vi "Intialize Shared Variable.vi"(8 "error in (no error)":errorcluster, 11 "Master Configuration":T1) -> (0 "error out":errorcluster)   [LabVIEW 2014]
uses:
  controls/Master Configuration.ctl
  controls/EPICS Configuration.ctl
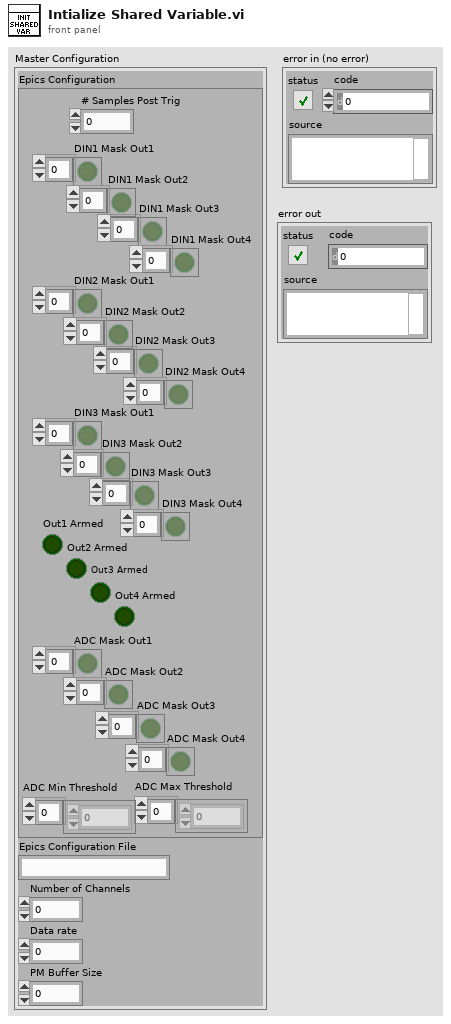
[diagram p1: front panel]
types:
  T1 = typedef "Master Configuration.ctl" = cluster{"Epics Configuration":T2, "Epics Configuration File":string, "Number of Channels":u8, "Data rate":u32, "PM Buffer Size":u32}
  T2 = typedef "EPICS Configuration.ctl" = cluster{"DIN1 Mask Out1":bool[], "# Samples Post Trig":u32, "ADC Mask Out1":bool[], "ADC Max Threshold":dbl[], "ADC Min Threshold":dbl[], "DIN1 Mask Out2":bool[], "DIN1 Mask Out3":bool[], "DIN1 Mask Out4":bool[], "Out3 Armed":bool, "Out1 Armed":bool, "Out4 Armed":bool, "Out2 Armed":bool, "DIN2 Mask Out1":bool[], "DIN2 Mask Out2":bool[], "DIN2 Mask Out3":bool[], "DIN2 Mask Out4":bool[], "DIN3 Mask Out1":bool[], "DIN3 Mask Out2":bool[], "DIN3 Mask Out3":bool[], "DIN3 Mask Out4":bool[], "ADC Mask Out2":bool[], "ADC Mask Out3":bool[], "ADC Mask Out4":bool[]}
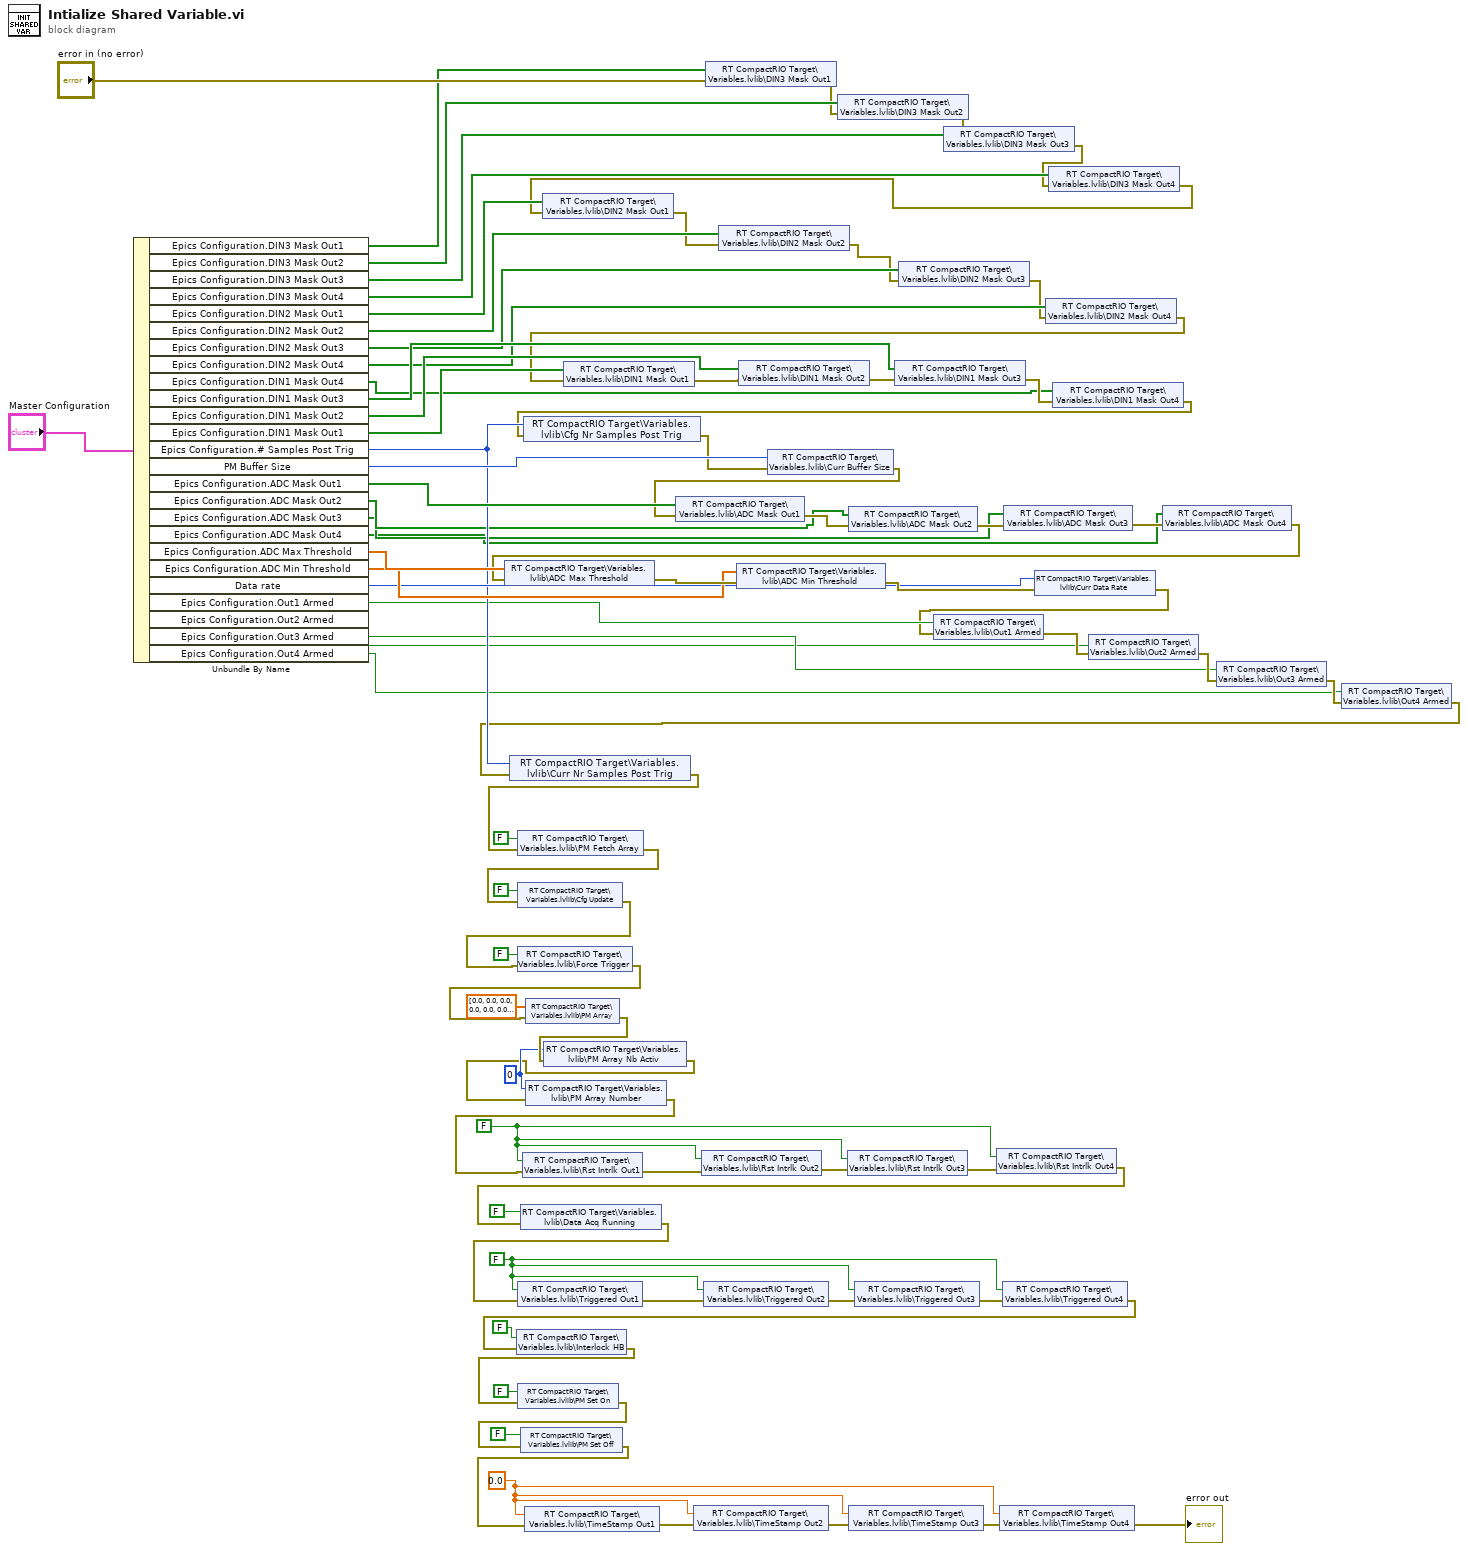
[diagram p0: block diagram]
diagram:
  w39 = 0.0 ("TimeStamp")
  w43 = FALSE ("Triggered")
  w48 = FALSE ("Reset Interlock")
  w2 = u8 0 ("PM Array Number")
  n1 = Unbundle By Name("Master Configuration") -> ("Epics Configuration.DIN3 Mask Out1"=w22:bool[], "Epics Configuration.DIN3 Mask Out2"=w23:bool[], "Epics Configuration.DIN3 Mask Out3"=w24:bool[], "Epics Configuration.DIN3 Mask Out4"=w25:bool[], "Epics Configuration.DIN2 Mask Out1"=w26:bool[], "Epics Configuration.DIN2 Mask Out2"=w27:bool[], "Epics Configuration.DIN2 Mask Out3"=w28:bool[], "Epics Configuration.DIN2 Mask Out4"=w29:bool[], "Epics Configuration.DIN1 Mask Out4"=w53:bool[], "Epics Configuration.DIN1 Mask Out3"=w54:bool[], "Epics Configuration.DIN1 Mask Out2"=w55:bool[], "Epics Configuration.DIN1 Mask Out1"=w79:bool[], "Epics Configuration.# Samples Post Trig"=w62:u32, "PM Buffer Size"=w64:u32, "Epics Configuration.ADC Mask Out1"=w75:bool[], "Epics Configuration.ADC Mask Out2"=w9:bool[], "Epics Configuration.ADC Mask Out3"=w8:bool[], "Epics Configuration.ADC Mask Out4"=w7:bool[], "Epics Configuration.ADC Max Threshold"=w73:dbl[], "Epics Configuration.ADC Min Threshold"=w72:dbl[], "Data rate"=w65:u32, "Epics Configuration.Out1 Armed"=w31:bool, "Epics Configuration.Out2 Armed"=w32:bool, "Epics Configuration.Out3 Armed"=w33:bool, "Epics Configuration.Out4 Armed"=w34:bool)
  n2 = shared-variable "RT CompactRIO Target\\Variables.lvlib\\DIN3 Mask Out1"(w22, error in="error in (no error)") -> (error out=w21:errorcluster)
  n3 = shared-variable "RT CompactRIO Target\\Variables.lvlib\\DIN3 Mask Out2"(w23, error in=w21) -> (error out=w20:errorcluster)
  n4 = shared-variable "RT CompactRIO Target\\Variables.lvlib\\DIN3 Mask Out3"(w24, error in=w20) -> (error out=w19:errorcluster)
  n5 = shared-variable "RT CompactRIO Target\\Variables.lvlib\\DIN3 Mask Out4"(w25, error in=w19) -> (error out=w18:errorcluster)
  n6 = shared-variable "RT CompactRIO Target\\Variables.lvlib\\DIN2 Mask Out1"(w26, error in=w18) -> (error out=w17:errorcluster)
  n7 = shared-variable "RT CompactRIO Target\\Variables.lvlib\\DIN2 Mask Out2"(w27, error in=w17) -> (error out=w16:errorcluster)
  n8 = shared-variable "RT CompactRIO Target\\Variables.lvlib\\DIN2 Mask Out3"(w28, error in=w16) -> (error out=w15:errorcluster)
  n9 = shared-variable "RT CompactRIO Target\\Variables.lvlib\\DIN2 Mask Out4"(w29, error in=w15) -> (error out=w14:errorcluster)
  n10 = shared-variable "RT CompactRIO Target\\Variables.lvlib\\DIN1 Mask Out1"(w79, error in=w14) -> (error out=w57:errorcluster)
  n11 = shared-variable "RT CompactRIO Target\\Variables.lvlib\\DIN1 Mask Out2"(w55, error in=w57) -> (error out=w59:errorcluster)
  n12 = shared-variable "RT CompactRIO Target\\Variables.lvlib\\DIN1 Mask Out3"(w54, error in=w59) -> (error out=w58:errorcluster)
  n13 = shared-variable "RT CompactRIO Target\\Variables.lvlib\\DIN1 Mask Out4"(w53, error in=w58) -> (error out=w56:errorcluster)
  n14 = shared-variable "RT CompactRIO Target\\Variables.lvlib\\Cfg Nr Samples Post Trig"(w62, error in=w56) -> (error out=w63:errorcluster)
  n15 = shared-variable "RT CompactRIO Target\\Variables.lvlib\\Curr Buffer Size"(w64, error in=w63) -> (error out=w4:errorcluster)
  n16 = shared-variable "RT CompactRIO Target\\Variables.lvlib\\ADC Mask Out1"(w75, error in=w4) -> (error out=w10:errorcluster)
  n17 = shared-variable "RT CompactRIO Target\\Variables.lvlib\\ADC Mask Out2"(w9, error in=w10) -> (error out=w13:errorcluster)
  n18 = shared-variable "RT CompactRIO Target\\Variables.lvlib\\ADC Mask Out3"(w8, error in=w13) -> (error out=w12:errorcluster)
  n19 = shared-variable "RT CompactRIO Target\\Variables.lvlib\\ADC Mask Out4"(w7, error in=w12) -> (error out=w11:errorcluster)
  n20 = shared-variable "RT CompactRIO Target\\Variables.lvlib\\ADC Max Threshold"(w73, error in=w11) -> (error out=w74:errorcluster)
  n21 = shared-variable "RT CompactRIO Target\\Variables.lvlib\\ADC Min Threshold"(w72, error in=w74) -> (error out=w71:errorcluster)
  n22 = shared-variable "RT CompactRIO Target\\Variables.lvlib\\Curr Data Rate"(w65, error in=w71) -> (error out=w5:errorcluster)
  n23 = shared-variable "RT CompactRIO Target\\Variables.lvlib\\Out1 Armed"(w31, error in=w5) -> (error out=w37:errorcluster)
  n24 = shared-variable "RT CompactRIO Target\\Variables.lvlib\\Out2 Armed"(w32, error in=w37) -> (error out=w36:errorcluster)
  n25 = shared-variable "RT CompactRIO Target\\Variables.lvlib\\Out3 Armed"(w33, error in=w36) -> (error out=w35:errorcluster)
  n26 = shared-variable "RT CompactRIO Target\\Variables.lvlib\\Out4 Armed"(w34, error in=w35) -> (error out=w6:errorcluster)
  n27 = shared-variable "RT CompactRIO Target\\Variables.lvlib\\Curr Nr Samples Post Trig"(w62, error in=w6) -> (error out=w61:errorcluster)
  n28 = shared-variable "RT CompactRIO Target\\Variables.lvlib\\PM Fetch Array"(FALSE ("PM Fetch Array"), error in=w61) -> (error out=w86:errorcluster)
  n29 = shared-variable "RT CompactRIO Target\\Variables.lvlib\\Cfg Update"(FALSE ("Cfg Update"), error in=w86) -> (error out=w83:errorcluster)
  n30 = shared-variable "RT CompactRIO Target\\Variables.lvlib\\Force Trigger"(FALSE ("Force Trigger"), error in=w83) -> (error out=w82:errorcluster)
  n31 = shared-variable "RT CompactRIO Target\\Variables.lvlib\\PM Array"(sgl[] [0.0, 0.0, 0.0, 0.0, 0.0, 0.0, 0.0, 0.0, 0.0, 0.0, 0.0, 0.0, 0.0, 0.0, 0.0, 0.0] ("PM Array"), error in=w82) -> (error out=w3:errorcluster)
  n32 = shared-variable "RT CompactRIO Target\\Variables.lvlib\\PM Array Nb Activ"(w2, error in=w3) -> (error out=w1:errorcluster)
  n33 = shared-variable "RT CompactRIO Target\\Variables.lvlib\\PM Array Number"(w2, error in=w1) -> (error out=w60:errorcluster)
  n34 = shared-variable "RT CompactRIO Target\\Variables.lvlib\\Rst Intrlk Out1"(w48, error in=w60) -> (error out=w50:errorcluster)
  n35 = shared-variable "RT CompactRIO Target\\Variables.lvlib\\Rst Intrlk Out2"(w48, error in=w50) -> (error out=w52:errorcluster)
  n36 = shared-variable "RT CompactRIO Target\\Variables.lvlib\\Rst Intrlk Out3"(w48, error in=w52) -> (error out=w51:errorcluster)
  n37 = shared-variable "RT CompactRIO Target\\Variables.lvlib\\Rst Intrlk Out4"(w48, error in=w51) -> (error out=w49:errorcluster)
  n38 = shared-variable "RT CompactRIO Target\\Variables.lvlib\\Data Acq Running"(FALSE ("Reset Interlock"), error in=w49) -> (error out=w77:errorcluster)
  n39 = shared-variable "RT CompactRIO Target\\Variables.lvlib\\Triggered Out1"(w43, error in=w77) -> (error out=w45:errorcluster)
  n40 = shared-variable "RT CompactRIO Target\\Variables.lvlib\\Triggered Out2"(w43, error in=w45) -> (error out=w47:errorcluster)
  n41 = shared-variable "RT CompactRIO Target\\Variables.lvlib\\Triggered Out3"(w43, error in=w47) -> (error out=w46:errorcluster)
  n42 = shared-variable "RT CompactRIO Target\\Variables.lvlib\\Triggered Out4"(w43, error in=w46) -> (error out=w44:errorcluster)
  n43 = shared-variable "RT CompactRIO Target\\Variables.lvlib\\Interlock HB"(FALSE ("Triggered"), error in=w44) -> (error out=w70:errorcluster)
  n44 = shared-variable "RT CompactRIO Target\\Variables.lvlib\\PM Set On"(FALSE ("PM Set On"), error in=w70) -> (error out=w68:errorcluster)
  n45 = shared-variable "RT CompactRIO Target\\Variables.lvlib\\PM Set Off"(FALSE ("PM Set On"), error in=w68) -> (error out=w66:errorcluster)
  n46 = shared-variable "RT CompactRIO Target\\Variables.lvlib\\TimeStamp Out1"(w39, error in=w66) -> (error out=w40:errorcluster)
  n47 = shared-variable "RT CompactRIO Target\\Variables.lvlib\\TimeStamp Out2"(w39, error in=w40) -> (error out=w42:errorcluster)
  n48 = shared-variable "RT CompactRIO Target\\Variables.lvlib\\TimeStamp Out3"(w39, error in=w42) -> (error out=w41:errorcluster)
  n49 = shared-variable "RT CompactRIO Target\\Variables.lvlib\\TimeStamp Out4"(w39, error in=w41) -> (error out=→"error out":errorcluster)
